vi "Set Heartbeats.vi"(8 "error in":errorcluster, 11 "CANopen Master in":refnum<class "CANopen Master.lvclass">) -> (0 "error out":errorcluster, 1 "Timed Outs?":bool[](array[boolean]), 2 "Node-IDs":u8[](array[numeric]), 3 "CANopen Master out":refnum<class "CANopen Master.lvclass">)   [LabVIEW 2024, in "CANopen Master.lvlib" / "CANopen Master.lvclass"]
uses:
  CANopen Master.lvclass
  CANopen Master.lvclass/CANopen Master.ctl
  Heartbeat/Heartbeat.lvclass
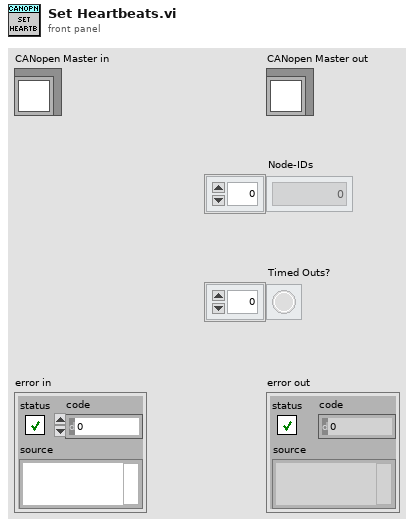
[diagram p1: front panel]
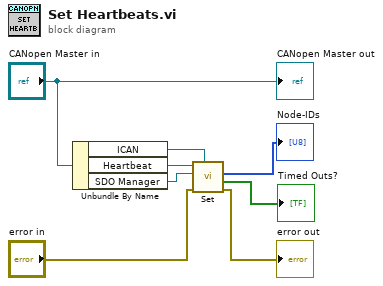
[diagram p0: block diagram]
diagram:
  n1 = Unbundle By Name("CANopen Master in") -> ("ICAN"=w1:refnum<class "ICAN.lvclass">, "Heartbeat"=w7:refnum<class "Heartbeat.lvclass">, "SDO Manager"=w4:refnum<class "SDO Manager.lvclass">)
  n2 = call "Set.vi"("ICAN"=w1, "Error In"="error in", "SDO Manager"=w4, "reference in"=w7) -> ("Error Out"=→"error out":errorcluster, "Timed Outs?"=→"Timed Outs?":bool[], "Node-IDs"=→"Node-IDs":u8[])  [unwired: 4 in, 1 out]
  "CANopen Master out" <- "CANopen Master in"
